vi "onHarvestPips.vi"(7 "TraceabilityMatrix in":refnum<class "TraceabilityMatrix.lvclass">, 11 "Pips":refnum<class "Pips.lvclass">) -> (0 "error out":errorcluster, 3 "Pips":refnum<class "Pips.lvclass">)   [LabVIEW 2021, in "Bananas.lvlib" / "TraceabilityMatrix.lvclass"]
uses:
  TraceabilityMatrix.lvclass
  Pips/Pips.lvclass
  Pips/statistics -- cluster.ctl
  Pips/pip_filter -- enum.ctl
  TraceabilityMatrix.lvclass/TraceabilityMatrix.ctl
panel:
  out "Blocked Tests":string[](array[string])
  out "Skipped Tests":string[](array[string])
  out "Failed Tests":string[](array[string])
  out "Statistics":T1 {"TestCases.BlockedPct" format="%.1g"; "TestCases.SkippedPct" format="%.1g"; "TestCases.FailedPct" format="%.1g"; "TestCases.NotImplementedPct" format="%.1g"; "TestCases.ImplementedPct" format="%.1g"; "TestCases.PassPct" format="%.1g"; "TestCases.FullyCoveredPct" format="%.1g"; "Requirements.NotCoveredPct" format="%.1g"; "Requirements.PartiallyCoveredPct" format="%.1g"; "Requirements.FullyCoveredPct" format="%.1g"}
  out "Nb Requirement with \"N\" Test Cases":cluster{i32[], i32[]}(graph)
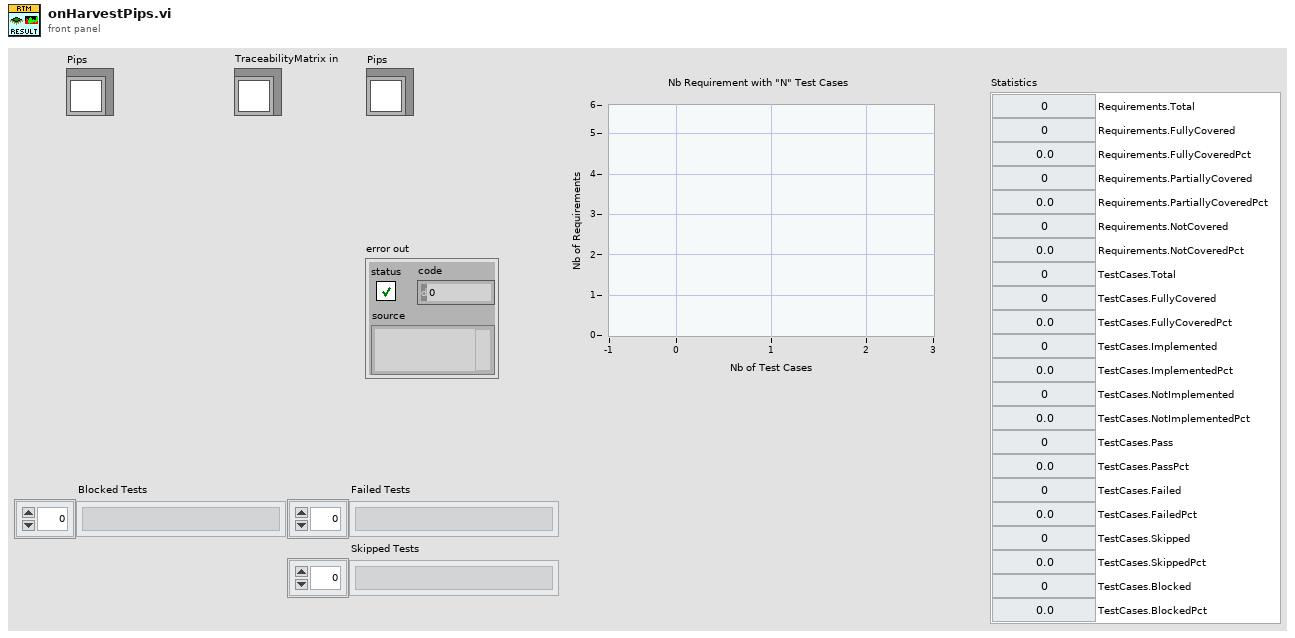
[diagram p1: front panel]
types:
  T1 = typedef "Bananas.lvlib/Pips.lvclass/statistics -- cluster.ctl" = cluster{"Requirements.Total":u32, "Requirements.FullyCovered":u32, "Requirements.FullyCoveredPct":dbl, "Requirements.PartiallyCovered":u32, "Requirements.PartiallyCoveredPct":dbl, "Requirements.NotCovered":u32, "Requirements.NotCoveredPct":dbl, "TestCases.Total":u32, "TestCases.FullyCovered":u32, "TestCases.FullyCoveredPct":dbl, "TestCases.Implemented":u32, "TestCases.ImplementedPct":dbl, "TestCases.NotImplemented":u32, "TestCases.NotImplementedPct":dbl, "TestCases.Pass":u32, "TestCases.PassPct":dbl, "TestCases.Failed":u32, "TestCases.FailedPct":dbl, "TestCases.Skipped":u32, "TestCases.SkippedPct":dbl, "TestCases.Blocked":u32, "TestCases.BlockedPct":dbl}
  T2 = typedef "Bananas.lvlib/Pips.lvclass/pip_filter -- enum.ctl" = enum16{"none", "passed", "skipped", "failed", "blocked", "implemented", "covered", "uncovered", "partially-covered"}
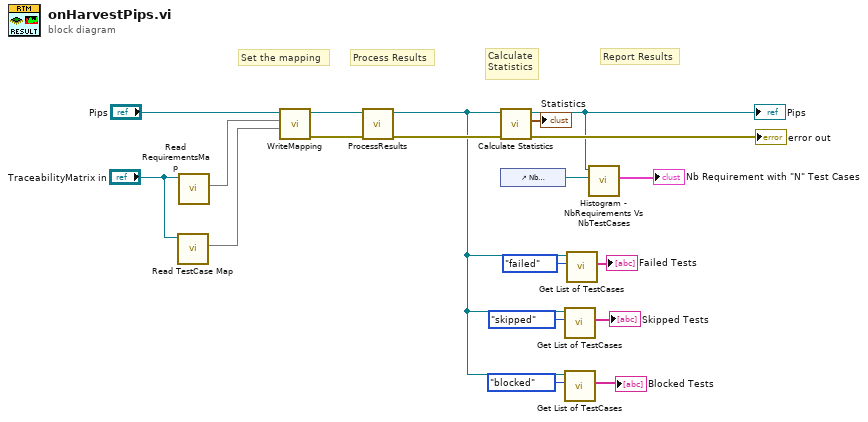
[diagram p0: block diagram]
diagram:
  # "Calculate\nStatistics"
  # "Report Results"
  # "Process Results"
  # "Set the mapping"
  n1 = call "Read TestCase Map.vi"("TraceabilityMatrix in"="TraceabilityMatrix in") -> ("TestCaseMap"=w16:map{string, set{string}})  [unwired: 9 in, 1 out]
  n2 = call "Read RequirementsMap.vi"("TraceabilityMatrix in"="TraceabilityMatrix in") -> ("RequirementMap"=w17:map{string, set{string}})  [unwired: 9 in, 1 out]
  n3 = call "WriteMapping.vi"("TestCaseMap"=w16, "RequirementMap"=w17, "Pips in"="Pips") -> ("error out"=w14:errorcluster, "Pips out"=w15:refnum<class "Pips.lvclass">)  [unwired: 7 in]
  n4 = call "ProcessResults.vi"("error in (no error)"=w14, "Pips in"=w15) -> ("error out"=w13:errorcluster, "Pips out"=w4:refnum<class "Pips.lvclass">)  [unwired: 8 in]
  n5 = call "Calculate Statistics.vi"("error in (no error)"=w13, "Pips in"=w4) -> ("error out"=→"error out":errorcluster, "Statistics"=→"Statistics":T1, "Pips out"=w11:refnum<class "Pips.lvclass">)  [unwired: 7 in]
  "Pips" <- w11
  n6 = control-ref of="Nb Requirement with \"N\" Test Cases"() -> (w10:refnum<vi>)
  n7 = call "Get List of TestCases.vi"("Filter"=pip_filter_--_enum."skipped", "Pips in"=w4) -> ("TestCases"=→"Skipped Tests":string[])  [unwired: 6 in, 3 out]
  n8 = call "Get List of TestCases.vi"("Filter"=pip_filter_--_enum."blocked", "Pips in"=w4) -> ("TestCases"=→"Blocked Tests":string[])  [unwired: 6 in, 3 out]
  n9 = call "Get List of TestCases.vi"("Filter"=pip_filter_--_enum."failed", "Pips in"=w4) -> ("TestCases"=→"Failed Tests":string[])  [unwired: 6 in, 3 out]
  n10 = call "Histogram - NbRequirements Vs NbTestCases.vi"("XYGraph Ref"=w10, "Pips in"=w11) -> ("Nb Requirement with \"N\" Test Cases"=→"Nb Requirement with \"N\" Test Cases":cluster{i32[], i32[]})  [unwired: 7 in, 2 out]
